vi "Update Graphs.vi"(0 "Select Graph":T10, 2 "appended array":refnum<vi>[](array[refnum]), 5 "ERD Graph  Ind 2":T9, 7 "ERD_Data_Bundled_In":T1, 11 "Error In":errorcluster) -> (3 "Temp":dbl(graph), 4 "Basket Speed":u16[][](graph), 6 "Tub Gallons":dbl(graph), 8 "Pressure 3":dbl(graph), 10 "Motor Current":dbl(graph), 12 "ERD 3":dbl(graph), 13 "ERD 2":dbl(graph), 14 "ERD 1":dbl(graph), 15 "Error Out":errorcluster)   [LabVIEW 2014]
doc: "This VI displays (makes visable) the corresponding graph based on user selection, as well as updates the values of the graphs with current data."
uses:
  type defs/Select Graph.ctl
  type defs/ERD_Data_Bundled.ctl
  type defs/ATC_Data.ctl
  type defs/Redundant.ctl
  type defs/Version.ctl
  type defs/Algorithms.ctl
  type defs/ERD_Always_Show.ctl
  type defs/Fault_Table_Info.ctl
  type defs/Cycle_Diag.ctl
panel:
  # "Wet Load Size"
  # "Dry Load Size"
  # "OOB"
  # "Software Version"
  # "Critical Version"
  # "Non-Critical"
  # "XML Crit Ver"
  # "XML Non-Crit"
  # "Daily Build"
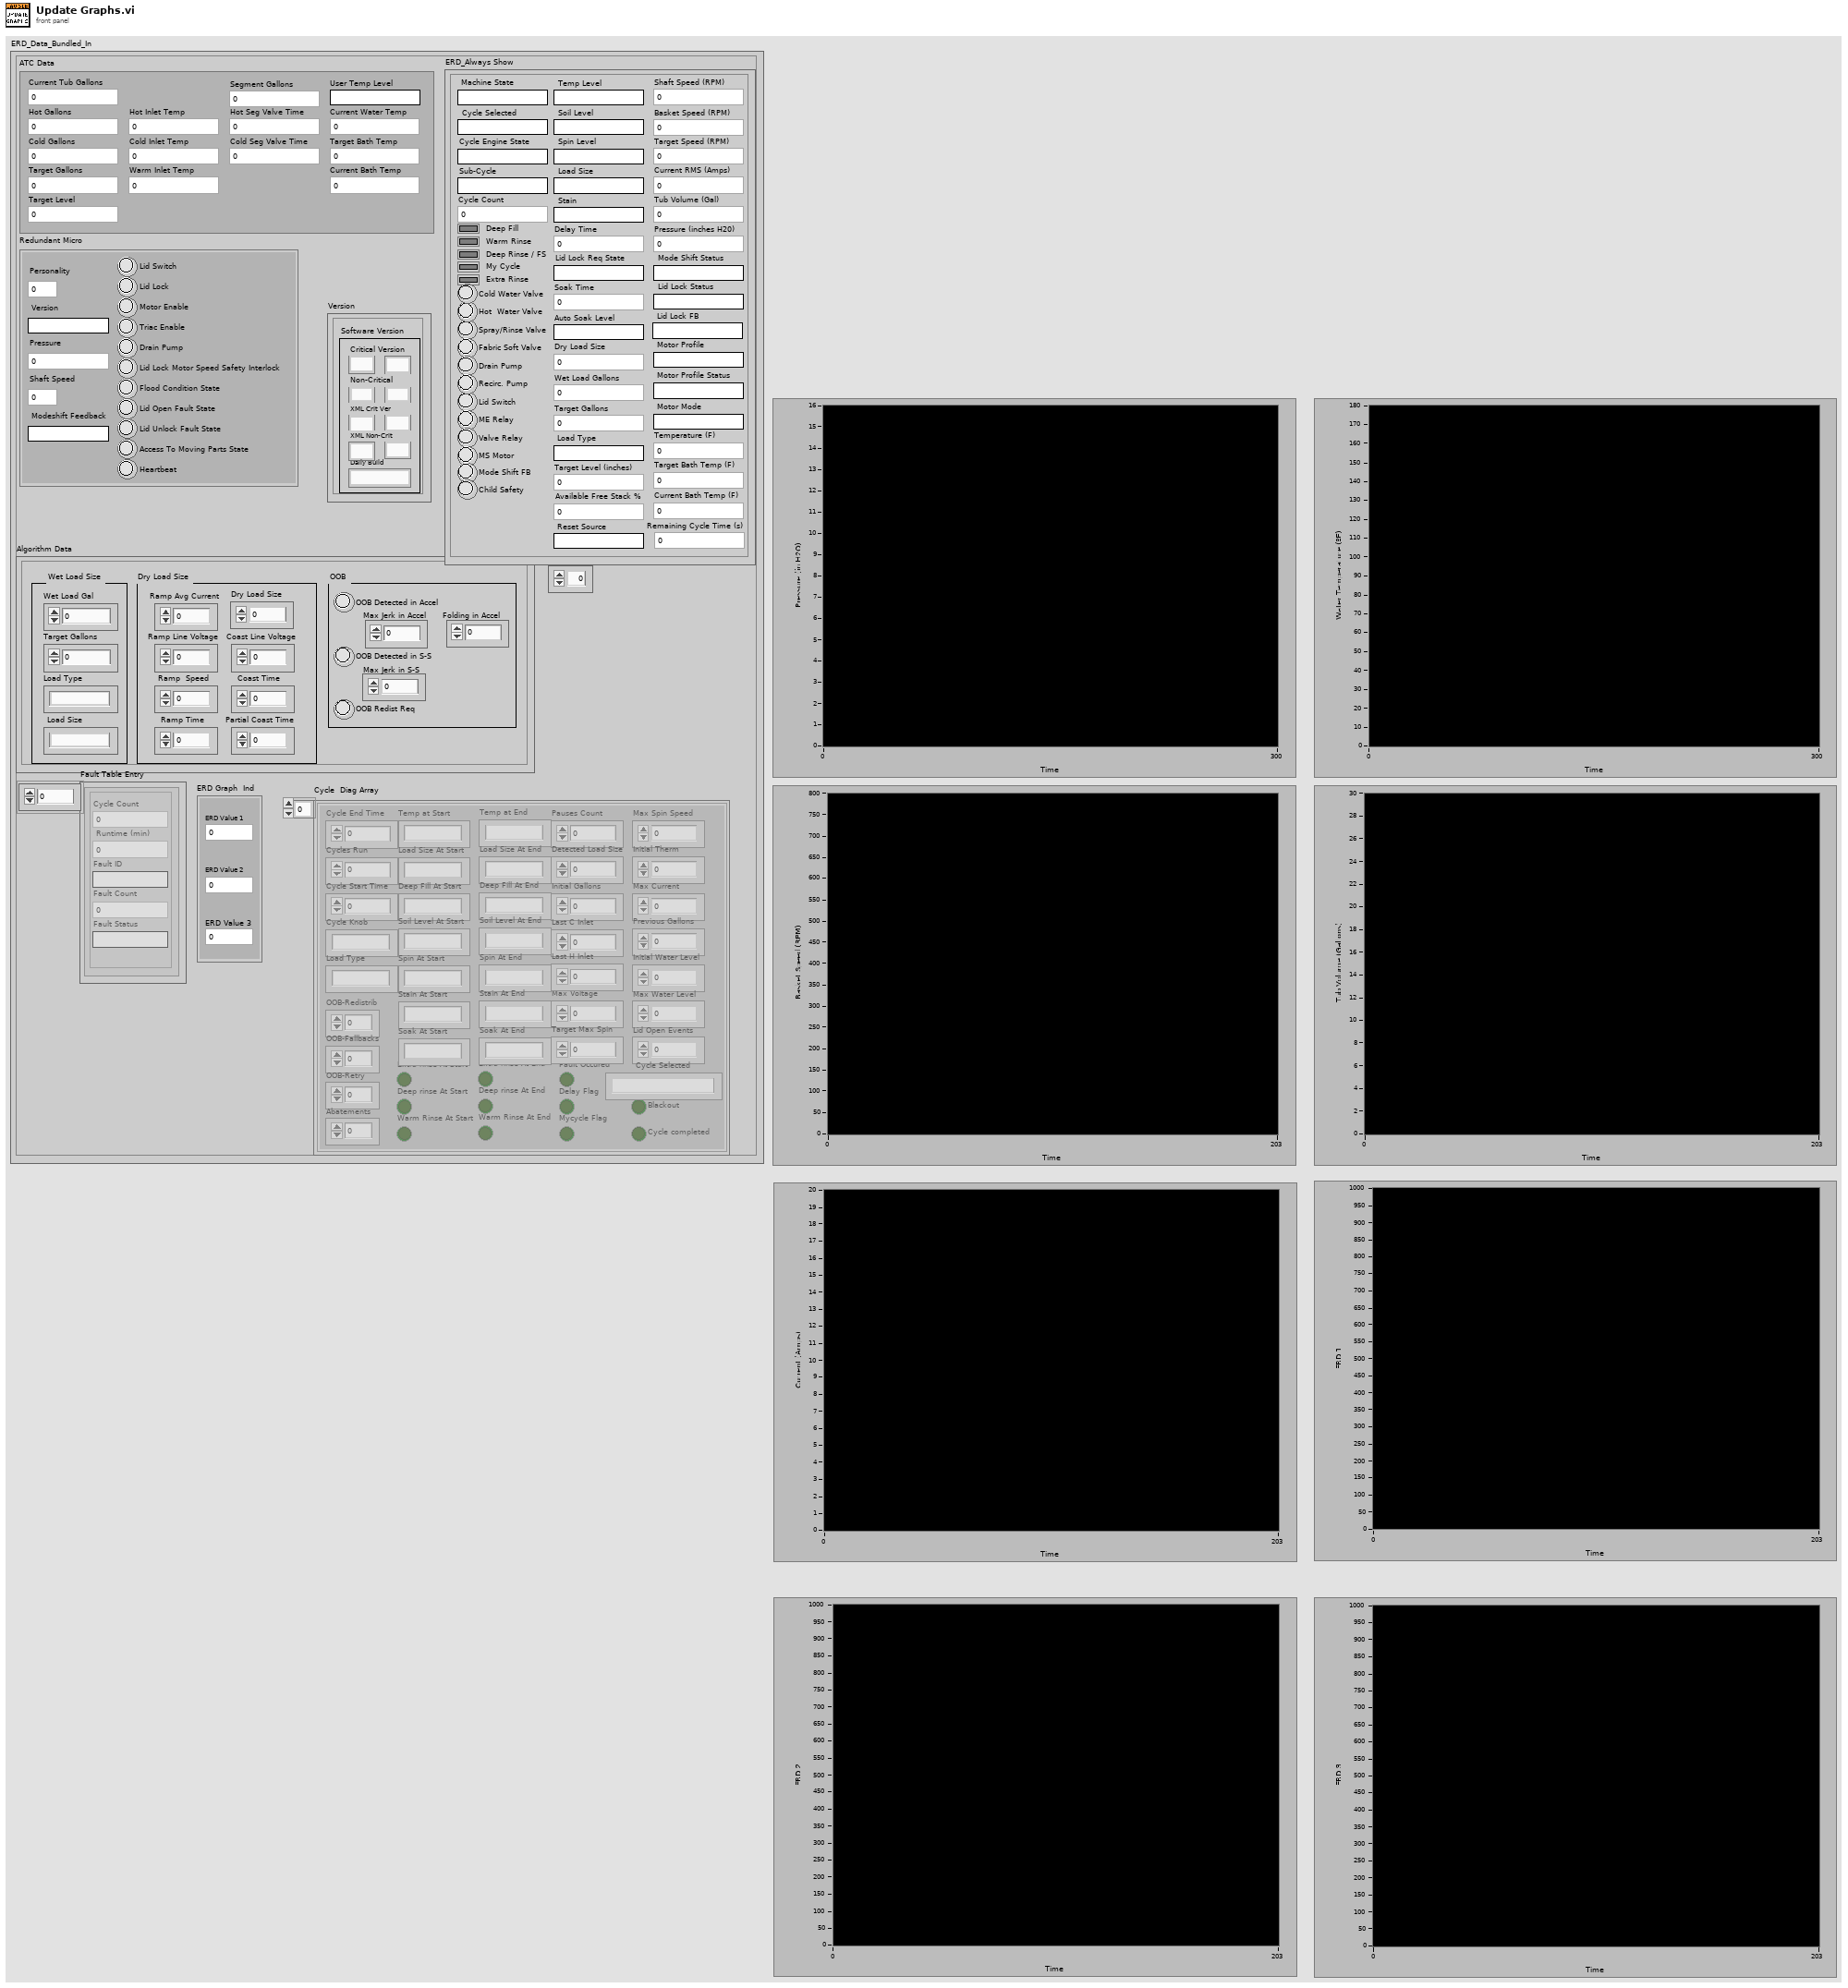
[diagram p1: front panel]
types:
  T1 = typedef "ERD_Data_Bundled.ctl" = cluster{"ATC Data":T2, "Redundant Micro":T3, "Version":T4, "Algorithm Data":T5, "ERD_Always Show":T6, "ERD Graph  Ind":cluster{"ERD Value 1":dbl, "ERD Value 2":dbl, "ERD Value 3":dbl}, "Personality Set":u8, "Fault Table Entry":T7[], "Cycle  Diag Array":T8[]}
  T2 = typedef "ATC_Data.ctl" = cluster{"Current Tub Gallons":dbl, "Hot Gallons":dbl, "Cold Gallons":dbl, "Target Gallons":dbl, "Current Water Temp":dbl, "Target Level":u32, "Target Bath Temp":dbl, "Current Bath Temp ":dbl, "Cold Inlet Temp":dbl, "Hot Inlet Temp":dbl, "Warm Inlet Temp":dbl, "Hot Seg Valve Time":u16, "Cold Seg Valve Time ":u16, "User Temp Level":string, "Segment Gallons":dbl}
  T3 = typedef "Redundant.ctl" = cluster{"Version":string, "Personality":u8, "Pressure ":dbl, "Shaft Speed":u16, "Modeshift Feedback":string, "Lid Switch":bool, "Lid Lock":bool, "Triac Enable":bool, "Drain Pump":bool, "Lid Lock Motor Speed Safety Interlock":bool, "Flood Condition State":bool, "Lid Open Fault State":bool, "Access To Moving Parts State":bool, "Heartbeat":bool, "Motor Enable":bool, "Lid Unlock Fault State":bool}
  T4 = typedef "Version.ctl" = cluster{"Critical Major":string, "Critical Minor":string, "Non-Critical Minor":string, "Non-Critical Major":string, "XML Crit Minor":string, "XMLCrit Major":string, "Daily Rev":string, "XML Non-crit Minor":string, "Xml Non-crit Major":string}
  T5 = typedef "Algorithms.ctl" = cluster{"Wet Load Gal":dbl, "Target Gallons":dbl, "Load Type":string, "Load Size":string, "Coast Time":u16, "Ramp Time":u16, "Ramp  Speed":u16, "Ramp Avg Current":dbl, "OOB Redist Req":bool, "OOB Detected in S-S":bool, "Folding in Accel":i32, "Max Jerk in Accel":i32, "Max Jerk in S-S":i32, "OOB Detected in Accel":bool, "Partial Coast Time":u16, "Dry Load Size":dbl, "Ramp Line Voltage ":dbl, "Coast Line Voltage":dbl}
  T6 = typedef "ERD_Always_Show.ctl" = cluster{"Basket Speed (RPM)":u16, "Machine State":string, "Tub Volume (Gal)":dbl, "Pressure (inches H20)":dbl, "Lid Switch ":bool, "Current RMS (Amps)":dbl, "Cycle Selected":string, "Lid Lock Status":string, "Mode Shift Status":string, "Spray/Rinse Valve":bool, "Fabric Soft Valve":bool, "Drain Pump":bool, "Recirc. Pump":bool, "Cycle Engine State":string, "Hot  Water Valve":bool, "Cold Water Valve":bool, "Motor Profile":string, "Motor Profile Status":string, "Motor Mode":string, "ME Relay":bool, "Cycle Count":u32, "Deep Rinse / FS":bool, "My Cycle":bool, "Soil Level":string, "Spin Level":string, "Stain":string, "Temp Level":string, "Load Size":string, "Delay Time":u16, "Soak Time":u16, "Deep Fill":bool, "Warm Rinse":bool, "Auto Soak Level":string, "Extra Rinse":bool, "Wet Load Gallons":dbl, "Target Gallons":dbl, "Sub-Cycle":string, "Load Type":string, "Target Level (inches)":u32, "Valve Relay":bool, "Dry Load Size":dbl, "Shaft Speed (RPM) ":u16, "MS Motor":bool, "Mode Shift FB":bool, "Target Bath Temp (F)":dbl, "Temperature (F)":dbl, "Current Bath Temp (F)":dbl, "Lid Lock FB":string, "Lid Lock Req State":string, "Remaining Cycle Time (s)":u32, "Available Free Stack %":u8, "Child Safety":bool, "Target Speed (RPM)":u16, "Reset Source":string}
  T7 = typedef "Fault_Table_Info.ctl" = cluster{"Cycle Count":u32, " Runtime (min) ":u32, "Fault Status":string, "Fault ID":string, "Fault Count":u16}
  T8 = typedef "Cycle_Diag.ctl" = cluster{"Cycle End Time":u32, "Cycles Run":u32, "Cycle Start Time":u32, "Cycle Knob":string, "Load Type":string, "OOB-Redistrib":u8, "OOB-Fallbacks":u8, "OOB-Retry":u8, "Temp at Start":string, "Load Size At Start":string, "Deep Fill At Start":string, "Soil Level At Start":string, "Spin At Start":string, "Extra rinse At Start":bool, "Deep rinse At Start":bool, "Stain At Start":string, "Soak At Start":string, "Warm Rinse At Start":bool, "Temp at End":string, "Load Size At End":string, "Deep Fill At End":string, "Soil Level At End":string, "Spin At End":string, "Extra rinse At End":bool, "Deep rinse At End":bool, "Stain At End":string, "Soak At End":string, "Warm Rinse At End":bool, "Pauses Count":u8, "Fault Occured":bool, "Delay Flag":bool, "Mycycle Flag":bool, "Blackout":bool, "Cycle completed":bool, "Detected Load Size":dbl, "Initial Gallons":dbl, "Last C Inlet ":dbl, "Max Voltage":dbl, "Target Max Spin":u16, "Max Spin Speed":u16, "Initial Therm":dbl, "Max Current":dbl, "Previous Gallons":dbl, "Initial Water Level":dbl, "Max Water Level":dbl, "Abatements ":u8, "Lid Open Events":u8, "Cycle Selected":string, "Last H Inlet ":dbl}
  T9 = cluster{"ERD Value 1":dbl, "ERD Value 2":dbl, "ERD Value 3":dbl}
  T10 = typedef "Select Graph.ctl" = enum16{"Temperature (F)", "Basket Speed (RPM)", "Tub Volume (Gal)", "Pressure (in H2O)", "Current RMS (Amps)", "ERD 1", "ERD 2", "ERD 3"}
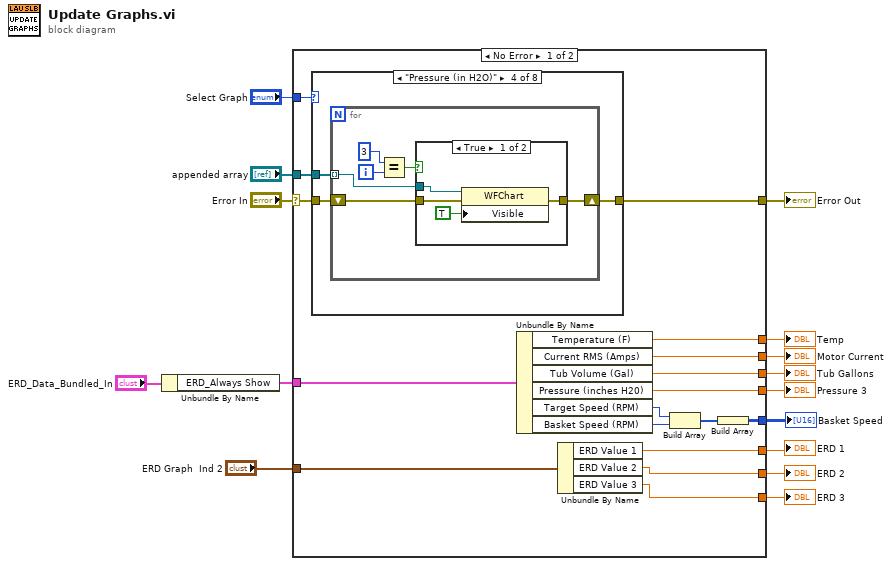
[diagram p0: block diagram]
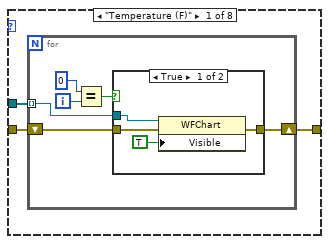
[diagram p2: hidden frame]
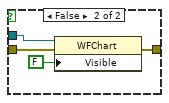
[diagram p3: hidden frame]
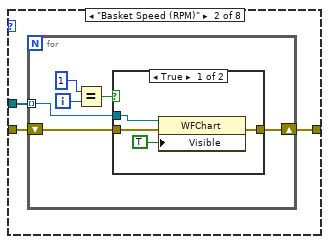
[diagram p4: hidden frame]
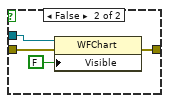
[diagram p5: hidden frame]
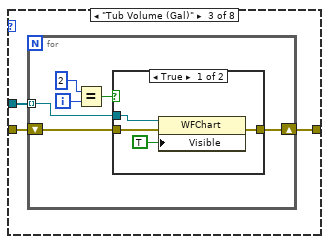
[diagram p6: hidden frame]
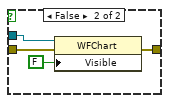
[diagram p7: hidden frame]
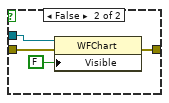
[diagram p8: hidden frame]
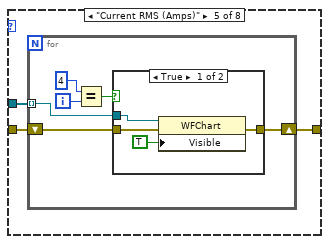
[diagram p9: hidden frame]
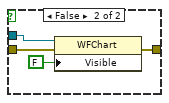
[diagram p10: hidden frame]
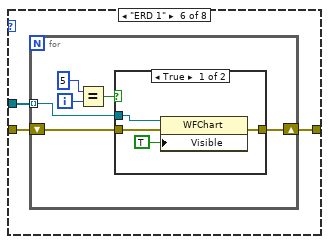
[diagram p11: hidden frame]
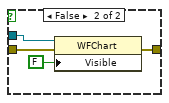
[diagram p12: hidden frame]
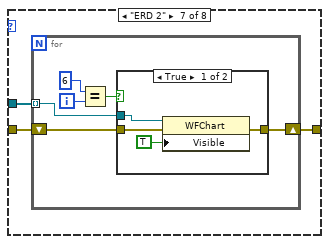
[diagram p13: hidden frame]
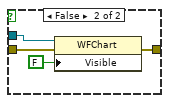
[diagram p14: hidden frame]
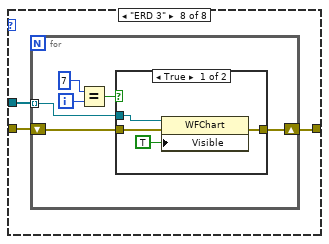
[diagram p15: hidden frame]
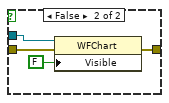
[diagram p16: hidden frame]
diagram:
  n1 = Unbundle By Name("ERD_Data_Bundled_In") -> ("ERD_Always Show"=w1:T6)
  n2 = case shown="No Error" "Error In" {
    selector: "Error In" -> [w29 w169]
    tunnel: [w28 w169] -> w14
    tunnel: w1 -> [w32 _]
    tunnel: "appended array" -> [w30 _]
    tunnel: "Select Graph" -> [w31 _]
    tunnel: [w27 _] -> w11
    tunnel: [w26 _] -> w10
    tunnel: [w25 _] -> w9
    tunnel: [w24 _] -> w8
    tunnel: "ERD Graph  Ind 2" -> [w23 _]
    tunnel: [w22 _] -> w6
    tunnel: [w21 _] -> w5
    tunnel: [w20 _] -> w4
    tunnel: [w16 _] -> w3
    frame No Error {
      n3 = case shown="\"Pressure (in H2O)\"" w31 {
        tunnel: w30 -> [w35 w52 w69 w86 w102 w119 w137 w152]
        tunnel: w29 -> [w34 w51 w68 w85 w103 w120 w136 w154]
        tunnel: [w33 w50 w67 w84 w101 w118 w135 w153] -> w28
        frame "Temperature (F)" {
          n4 = for {
            tunnel: w35 -> [w41] mode=indexing
            shift-right: [w39] -> w33
            shift-left: w34 -> [w40]
            i -> [w38]
            n5 = Equal?(x=0 ("index"), y=w38) -> (x = y?=w36:bool)
            n6 = case shown="True" w36 {
              tunnel: w41 -> [w45 w49]
              tunnel: w40 -> [w43 w47]
              tunnel: [w42 w46] -> w39
              frame True {
                n7 = property class="WFChart"(reference=w45, error in=w43, "Visible"=TRUE) -> (error out=w42:errorcluster)  [unwired: 1 out]
              }
              frame False {
                n8 = property class="WFChart"(reference=w49, error in=w47, "Visible"=FALSE) -> (error out=w46:errorcluster)  [unwired: 1 out]
              }
            }
          }
        }
        frame "Basket Speed (RPM)" {
          n9 = for {
            tunnel: w52 -> [w58] mode=indexing
            shift-right: [w56] -> w50
            shift-left: w51 -> [w57]
            i -> [w55]
            n10 = Equal?(x=1 ("index"), y=w55) -> (x = y?=w53:bool)
            n11 = case shown="True" w53 {
              tunnel: w58 -> [w62 w66]
              tunnel: w57 -> [w60 w64]
              tunnel: [w59 w63] -> w56
              frame True {
                n12 = property class="WFChart"(reference=w62, error in=w60, "Visible"=TRUE) -> (error out=w59:errorcluster)  [unwired: 1 out]
              }
              frame False {
                n13 = property class="WFChart"(reference=w66, error in=w64, "Visible"=FALSE) -> (error out=w63:errorcluster)  [unwired: 1 out]
              }
            }
          }
        }
        frame "Tub Volume (Gal)" {
          n14 = for {
            tunnel: w69 -> [w75] mode=indexing
            shift-right: [w73] -> w67
            shift-left: w68 -> [w74]
            i -> [w72]
            n15 = Equal?(x=2 ("index"), y=w72) -> (x = y?=w70:bool)
            n16 = case shown="True" w70 {
              tunnel: w75 -> [w79 w83]
              tunnel: w74 -> [w77 w81]
              tunnel: [w76 w80] -> w73
              frame True {
                n17 = property class="WFChart"(reference=w79, error in=w77, "Visible"=TRUE) -> (error out=w76:errorcluster)  [unwired: 1 out]
              }
              frame False {
                n18 = property class="WFChart"(reference=w83, error in=w81, "Visible"=FALSE) -> (error out=w80:errorcluster)  [unwired: 1 out]
              }
            }
          }
        }
        frame "Pressure (in H2O)" {
          n19 = for {
            tunnel: w86 -> [w92] mode=indexing
            shift-right: [w90] -> w84
            shift-left: w85 -> [w91]
            i -> [w89]
            n20 = Equal?(x=3 ("index"), y=w89) -> (x = y?=w87:bool)
            n21 = case shown="True" w87 {
              tunnel: w92 -> [w96 w100]
              tunnel: w91 -> [w94 w98]
              tunnel: [w93 w97] -> w90
              frame True {
                n22 = property class="WFChart"(reference=w96, error in=w94, "Visible"=TRUE) -> (error out=w93:errorcluster)  [unwired: 1 out]
              }
              frame False {
                n23 = property class="WFChart"(reference=w100, error in=w98, "Visible"=FALSE) -> (error out=w97:errorcluster)  [unwired: 1 out]
              }
            }
          }
        }
        frame "Current RMS (Amps)" {
          n24 = for {
            tunnel: w102 -> [w109] mode=indexing
            shift-right: [w107] -> w101
            shift-left: w103 -> [w108]
            i -> [w106]
            n25 = Equal?(x=4 ("index"), y=w106) -> (x = y?=w104:bool)
            n26 = case shown="True" w104 {
              tunnel: w109 -> [w113 w117]
              tunnel: w108 -> [w111 w115]
              tunnel: [w110 w114] -> w107
              frame True {
                n27 = property class="WFChart"(reference=w113, error in=w111, "Visible"=TRUE) -> (error out=w110:errorcluster)  [unwired: 1 out]
              }
              frame False {
                n28 = property class="WFChart"(reference=w117, error in=w115, "Visible"=FALSE) -> (error out=w114:errorcluster)  [unwired: 1 out]
              }
            }
          }
        }
        frame "ERD 1" {
          n29 = for {
            tunnel: w119 -> [w126] mode=indexing
            shift-right: [w124] -> w118
            shift-left: w120 -> [w125]
            i -> [w123]
            n30 = Equal?(x=5 ("index"), y=w123) -> (x = y?=w121:bool)
            n31 = case shown="True" w121 {
              tunnel: w126 -> [w130 w134]
              tunnel: w125 -> [w128 w132]
              tunnel: [w127 w131] -> w124
              frame True {
                n32 = property class="WFChart"(reference=w130, error in=w128, "Visible"=TRUE) -> (error out=w127:errorcluster)  [unwired: 1 out]
              }
              frame False {
                n33 = property class="WFChart"(reference=w134, error in=w132, "Visible"=FALSE) -> (error out=w131:errorcluster)  [unwired: 1 out]
              }
            }
          }
        }
        frame "ERD 2" {
          n34 = for {
            tunnel: w137 -> [w143] mode=indexing
            shift-right: [w141] -> w135
            shift-left: w136 -> [w142]
            i -> [w140]
            n35 = Equal?(x=6 ("index"), y=w140) -> (x = y?=w138:bool)
            n36 = case shown="True" w138 {
              tunnel: w143 -> [w147 w151]
              tunnel: w142 -> [w145 w149]
              tunnel: [w144 w148] -> w141
              frame True {
                n37 = property class="WFChart"(reference=w147, error in=w145, "Visible"=TRUE) -> (error out=w144:errorcluster)  [unwired: 1 out]
              }
              frame False {
                n38 = property class="WFChart"(reference=w151, error in=w149, "Visible"=FALSE) -> (error out=w148:errorcluster)  [unwired: 1 out]
              }
            }
          }
        }
        frame "ERD 3" {
          n39 = for {
            tunnel: w152 -> [w160] mode=indexing
            shift-right: [w158] -> w153
            shift-left: w154 -> [w159]
            i -> [w157]
            n40 = Equal?(x=7 ("index"), y=w157) -> (x = y?=w155:bool)
            n41 = case shown="True" w155 {
              tunnel: w160 -> [w164 w168]
              tunnel: w159 -> [w162 w166]
              tunnel: [w161 w165] -> w158
              frame True {
                n42 = property class="WFChart"(reference=w164, error in=w162, "Visible"=TRUE) -> (error out=w161:errorcluster)  [unwired: 1 out]
              }
              frame False {
                n43 = property class="WFChart"(reference=w168, error in=w166, "Visible"=FALSE) -> (error out=w165:errorcluster)  [unwired: 1 out]
              }
            }
          }
        }
      }
      n44 = Unbundle By Name(w32) -> ("Temperature (F)"=w27:dbl, "Current RMS (Amps)"=w26:dbl, "Tub Volume (Gal)"=w25:dbl, "Pressure (inches H20)"=w24:dbl, "Target Speed (RPM)"=w19:u16, "Basket Speed (RPM)"=w18:u16)
      n45 = Unbundle By Name(w23) -> ("ERD Value 1"=w22:dbl, "ERD Value 2"=w21:dbl, "ERD Value 3"=w20:dbl)
      n46 = Build Array(w19, w18) -> (w17:u16[])
      n47 = Build Array(w17) -> (w16:u16[][])
    }
    frame Error {
    }
  }
  "Error Out" <- w14
  "Temp" <- w11
  "Basket Speed" <- w3
  "Motor Current" <- w10
  "Tub Gallons" <- w9
  "Pressure 3" <- w8
  "ERD 1" <- w6
  "ERD 2" <- w5
  "ERD 3" <- w4
